vi "Channel 0 Timer And Data Read (SubVI).vi"(0 "N":i32, 5 "BoardHandle in":T1, 7 "Channel # in":i32, 9 "dt (s) in":i32, 11 "error in (no error)":errorcluster) -> (1 "Actual Voltage Level (V)":dbl format="%#_13g", 2 "Power Supply Trip":bool, 3 "Actual Current Limit (nA)":dbl format="%#_13g", 4 "OVV?":bool=TRUE, 6 "Channel # out 2":i32, 8 "OVC?":bool=TRUE, 10 "Array":dbl[](array[numeric]), 12 "dt (s) out":i32, 13 "Time Left (s)":dbl, 14 "BoardHandle out 2":T1, 15 "error out":errorcluster)   [LabVIEW 2020]
uses:
  <instrlib>/CAEN PSM/CAEN PSM.lvlib
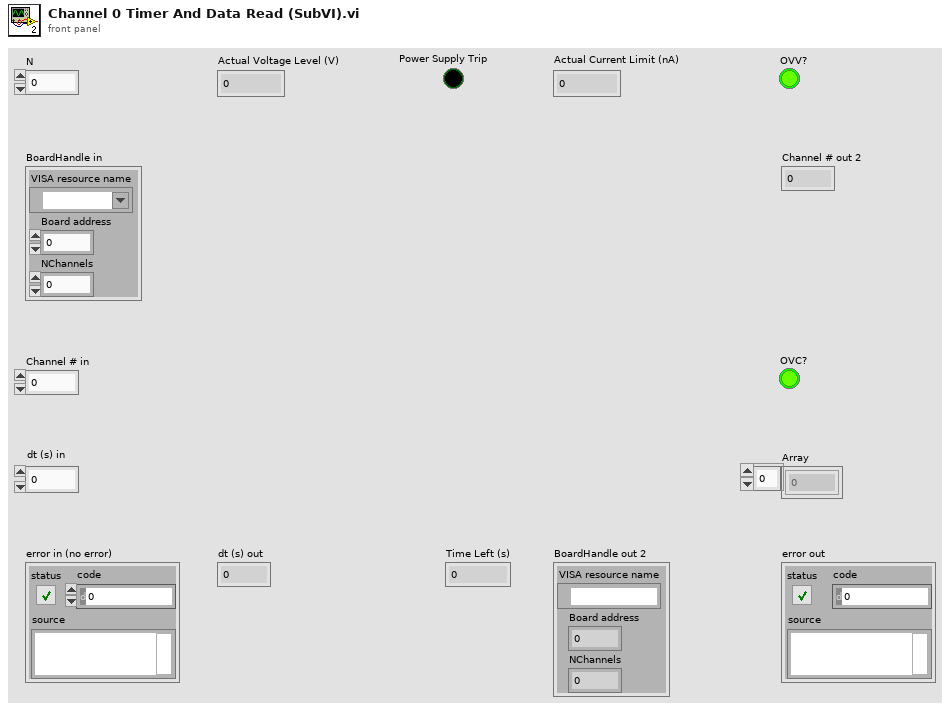
[diagram p1: front panel]
types:
  T1 = cluster{"VISA resource name":refnum<visa-resource-name>, "Board address":u8, "NChannels":u8}
  T2 = cluster{"ON":bool, "RUP":bool, "RDW":bool, "OVC":bool, "OVV":bool, "UNV":bool, "MAXV":bool, "TRIP":bool, "OVP":bool, "OVT":bool, "DIS":bool, "KILL":bool, "ILK":bool, "NOCAL":bool}[]
  T3 = cluster{"ON":bool, "RUP":bool, "RDW":bool, "OVC":bool, "OVV":bool, "UNV":bool, "MAXV":bool, "TRIP":bool, "OVP":bool, "OVT":bool, "DIS":bool, "KILL":bool, "ILK":bool, "NOCAL":bool}
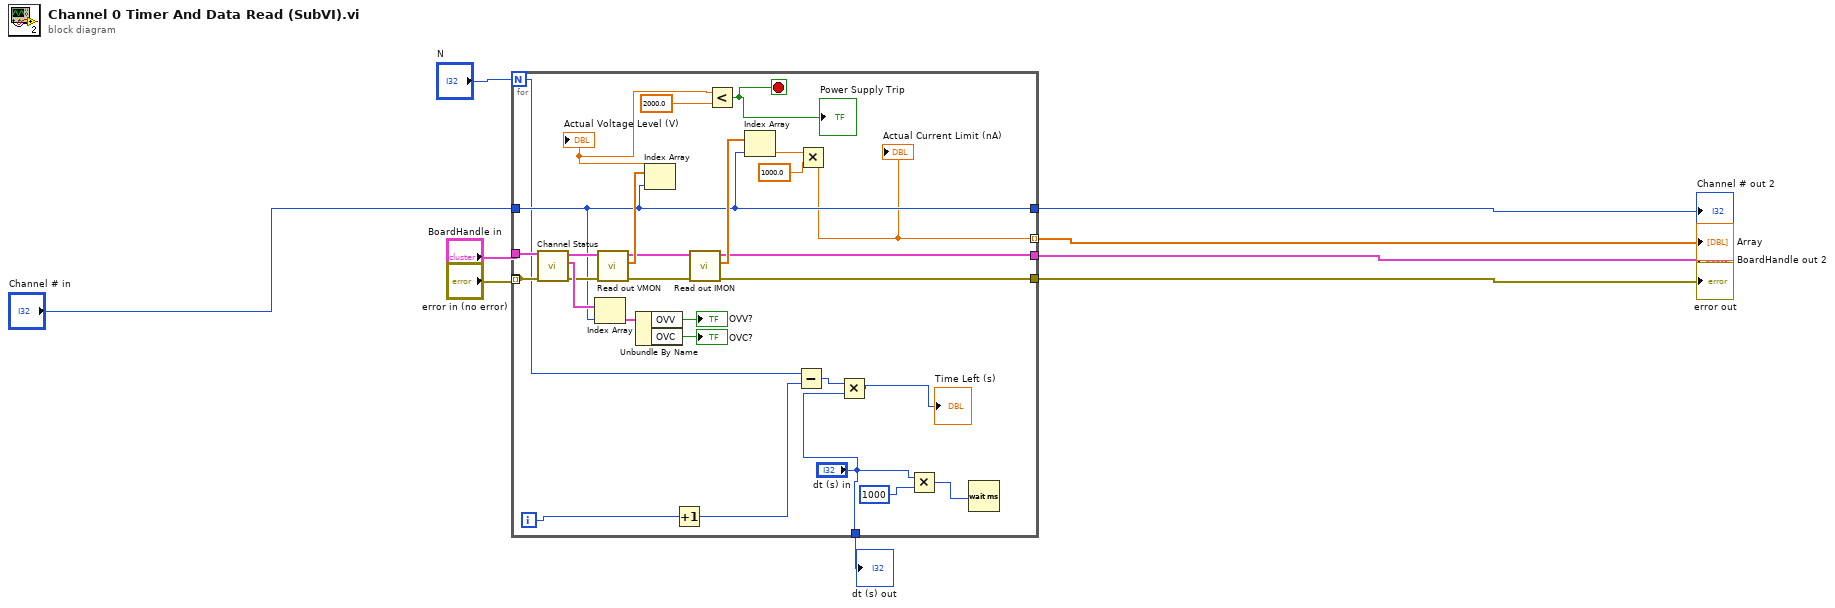
[diagram p0: block diagram]
diagram:
  n1 = for {
    N: "N" -> [w18]
    tunnel: "error in (no error)" -> [w25]
    tunnel: "Channel # in" -> [w26]
    tunnel: [w28] -> w2
    tunnel: [w27] -> w3
    tunnel: [w19] -> w8 mode=indexing
    tunnel: [w26] -> w4
    tunnel: "BoardHandle in" -> [w22]
    tunnel: [w25] -> _ mode=indexing
    tunnel: ["dt (s) in"] -> w9
    i -> [w15]
    stop <- w13 stop-if-true
    n2 = call <instrlib>:"Channel Status.vi"("error in (no error)"=w25, "BoardHandle"=w22) -> ("error out"=w34:errorcluster, "Channel Status Array"=w38:T2, "BoardHandle out"=w33:T1)  [unwired: 7 in]
    n3 = Index Array(array=w38, index=w26) -> (element=w37:T3)
    n4 = call <instrlib>:"Read out VMON.vi"("error in (no error)"=w34, "BoardHandle"=w33) -> ("error out"=w30:errorcluster, "VMon values (V)"=w32:dbl[], "BoardHandle out"=w31:T1)  [unwired: 7 in]
    n5 = Unbundle By Name(w37) -> ("OVV"=→"OVV?":bool, "OVC"=→"OVC?":bool)
    n6 = Index Array(array=w32, index=w26) -> (element=w12:dbl)
    "Actual Voltage Level (V)" <- w12
    n7 = Increment(x=w15) -> (x+1=w14:i32)
    n8 = call <instrlib>:"Read out IMON.vi"("error in (no error)"=w30, "BoardHandle"=w31) -> ("error out"=w27:errorcluster, "IMon values (uA)"=w29:dbl[], "BoardHandle out"=w28:T1)  [unwired: 6 in, 1 out]
    n9 = Less?(x=w12, y=2000.0) -> (x < y?=w13:bool)
    "Power Supply Trip" <- w13
    n10 = Index Array(array=w29, index=w26) -> (element=w21:dbl)
    n11 = Subtract(x=w18, y=w14) -> (x-y=w17:i32)
    n12 = Multiply(x=w21, y=1000.0) -> (x*y=w19:dbl)
    "Actual Current Limit (nA)" <- w19
    n13 = Multiply(x=w17, y="dt (s) in") -> (x*y=→"Time Left (s)":i32)
    n14 = Multiply(x="dt (s) in", y=1000) -> (x*y=w24:i32)
    n15 = Wait (ms)(milliseconds to wait=w24) -> ()  [unwired: 1 out]
  }
  "dt (s) out" <- w9
  "Array" <- w8
  "Channel # out 2" <- w4
  "error out" <- w3
  "BoardHandle out 2" <- w2
